vi "Test Old Report is Not Overwritten on Second Test Start.vi"(8 "error in (no error)":errorcluster, 11 "XML Report Test in":refnum<class "Report Generator Test.lvclass">) -> (0 "error out":errorcluster, 3 "XML Report Test out":refnum<class "Report Generator Test.lvclass">)   [LabVIEW 2020, in "Report Generator Test.lvclass"]
uses:
  Report Generator Test.lvclass
  C:/Program Files (x86)/National Instruments/LabVIEW 2020/vi.lib/Astemes/LUnit/Test Case.lvclass
  Report Generator Test.lvclass/Report Generator Test.ctl
  <vilib>/Astemes/LUnit/Test Case.lvclass/Test Case.ctl
  538b6b46-2778-4cbc-9a22-6f9245e30f78.vi
  <vilib>/Astemes/LUnit/Core/LUnit Test Case/Private/Append Fail Result.vi
  <vilib>/Astemes/LUnit/Core/LUnit Test Case/Private/Append Pass Result.vi
  538b6b46-2778-4cbc-9a22-6f9245e30f78.vi/4479f1b4-f4e5-41cd-8a07-3589632eefcf.vi
  <vilib>/Astemes/LUnit/Core/LUnit Test Case/Private/Run In UI.vi
  Test Doubles/Mock Report/Mock Report.lvclass
  C:/git/astemes-lunit/source/Plugins/Report/Report.lvclass
  source/Plugins/Report/Report.lvclass
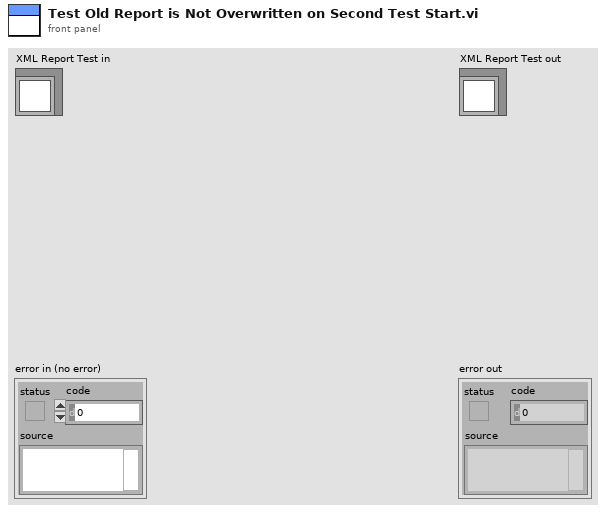
[diagram p1: front panel]
types:
  T1 = enum16{"open", "replace", "create", "open or create", "replace or create", "replace or create with confirmation"}
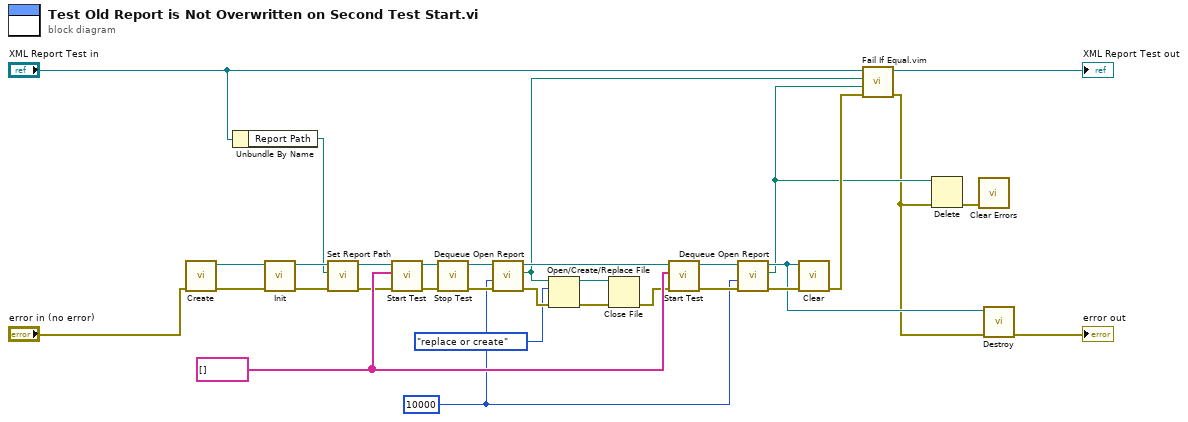
[diagram p0: block diagram]
diagram:
  w9 = 10000 ("timeout in ms (0)")
  w18 = string[] [] ("Tests")
  n1 = call "Create.vi"("error in (no error)"="error in (no error)") -> ("error out"=w25:errorcluster, "Mock Report Out"=w27:refnum<class "Mock Report.lvclass">)  [unwired: 9 in]
  n2 = Unbundle By Name("XML Report Test in") -> ("Report Path"=w10:path)
  n3 = call-dynamic "Init.vi"("error in (no error)"=w25, "Mock Report In"=w27) -> ("error out"=w31:errorcluster, "Mock Report Out"=w13:refnum<class "Mock Report.lvclass">)  [unwired: 8 in]
  n4 = call "Set Report Path.vi"("error in (no error)"=w31, "Report Path"=w10, "Report In"=w13) -> ("error out"=w14:errorcluster, "Report Out"=w12:refnum<class "Mock Report.lvclass">)  [unwired: 7 in]
  n5 = call-dynamic "Start Test.vi"("error in (no error)"=w14, "Tests"=w18, "XML Report in"=w12) -> ("error out"=w30:errorcluster, "XML Report out"=w21:refnum<class "Mock Report.lvclass">)  [unwired: 7 in]
  n6 = call-dynamic "Stop Test.vi"("error in (no error)"=w30, "XML Report in"=w21) -> ("error out"=w22:errorcluster, "XML Report out"=w16:refnum<class "Mock Report.lvclass">)  [unwired: 8 in]
  n7 = call "Dequeue Open Report.vi"("error in (no error)"=w22, "timeout in ms (0)"=w9, "Mock Report In"=w16) -> ("error out"=w17:errorcluster, "path"=w2:path, "Mock Report Out"=w15:refnum<class "Mock Report.lvclass">)  [unwired: 5 in, 1 out]
  n8 = Open/Create/Replace File(file path (use dialog)=w2, error in=w17, operation (0:open)=T1."replace or create") -> (refnum out=w3:refnum<file>, error out=w5:errorcluster)  [unwired: 3 in, 1 out]
  n9 = Close File(refnum=w3, error in=w5) -> (error out=w4:errorcluster)  [unwired: 1 out]
  n10 = call-dynamic "Start Test.vi"("error in (no error)"=w4, "Tests"=w18, "XML Report in"=w15) -> ("error out"=w20:errorcluster, "XML Report out"=w19:refnum<class "Mock Report.lvclass">)  [unwired: 7 in]
  n11 = call "Dequeue Open Report.vi"("error in (no error)"=w20, "timeout in ms (0)"=w9, "Mock Report In"=w19) -> ("error out"=w29:errorcluster, "path"=w8:path, "Mock Report Out"=w23:refnum<class "Mock Report.lvclass">)  [unwired: 5 in, 1 out]
  n12 = call-dynamic "Clear.vi"("error in (no error)"=w29, "XML Report in"=w23) -> ("error out"=w28:errorcluster)  [unwired: 9 in]
  n13 = call "Fail If Equal.vim"("error in (no error)"=w28, "Actual"=w8, "Unexpected"=w2, "LUnit Test Case In"="XML Report Test in") -> ("error out"=w7:errorcluster, "LUnit Test Case Out"=→"XML Report Test out":refnum<class "Report Generator Test.lvclass">)  [unwired: 6 in]
  n14 = Delete(path (use dialog)=w8, error in=w7) -> (error out=w6:errorcluster)  [unwired: 3 in, 2 out]
  n15 = call <vilib>:"Clear Errors.vi"("error in (no error)"=w6) -> ()  [unwired: 5 in, 2 out]
  n16 = call "Destroy.vi"("error in (no error)"=w7, "Mock Report In"=w23) -> ("error out"=→"error out":errorcluster)  [unwired: 9 in]
